vi "GetUnmodifiedSerializableData.vi"(8 "error in (no error)":errorcluster, 11 "BlueSerializable in":refnum<class "BlueSerializable.lvclass">) -> (0 "error out":errorcluster, 2 "SerializableData (parent,child)":variant[](array[variant]), 3 "BlueSerializable out":refnum<class "BlueSerializable.lvclass">)   [LabVIEW 2020, in "BlueSerialization.lvlib" / "BlueSerializer.lvclass"]
uses:
  BlueSerializer.lvclass
  BlueSerializable/BlueSerializable.lvclass
  SerializeOptionsPayload.ctl
  SerializeOptions.ctl
  ClassNameCacheMap.ctl
  ClassNameObj.ctl
  GetSerializableDataAction.ctl
  Support/GetSerializableDataCluster.ctl
  Support/GetSerializableDataClusterClass.ctl
  Support/SerializableDataGetDataAction.ctl
  ClassNameAndVersion.ctl
  <vilib>/Utility/EditLVLibs/LibVersion.ctl
  <vilib>/Utility/EditLVLibs/Edit LVLibs.lvlib
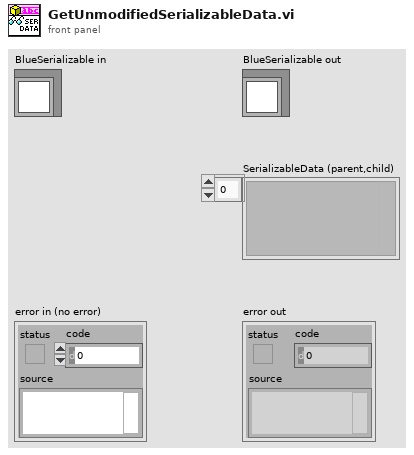
[diagram p1: front panel]
types:
  T1 = typedef "BlueSerialization.lvlib/BlueSerializer.lvclass/SerializeOptionsPayload.ctl" = cluster{"Serialize":T2, "ClassName Cache":refnum<data-value>}
  T2 = typedef "BlueSerialization.lvlib/BlueSerializer.lvclass/SerializeOptions.ctl" = cluster{"serialize non-BlueSerializable objects as hex?":bool, "slice objects per SetSerializeSliceClass.vi?":bool}
  T3 = typedef "BlueSerialization.lvlib/BlueSerializer.lvclass/GetSerializableDataAction.ctl" = enum16{"Ready For Flatten", "Unmodified Data Access"}
  T4 = typedef "BlueSerialization.lvlib/BlueSerializer.lvclass/GetSerializableDataCluster.ctl" = cluster{"Run-Mode":T3, "ClassOps":T5[], "Data":variant[], "PlaceholderData?":bool[]}
  T5 = typedef "BlueSerialization.lvlib/BlueSerializer.lvclass/GetSerializableDataClusterClass.ctl" = cluster{"Action":T6, "Class":T7}
  T6 = typedef "BlueSerialization.lvlib/BlueSerializer.lvclass/SerializableDataGetDataAction.ctl" = enum16{"Add Class", "Drop Class"}
  T7 = typedef "BlueSerialization.lvlib/BlueSerializer.lvclass/ClassNameAndVersion.ctl" = cluster{"class name":string, "Class Version":T8}
  T8 = typedef "Edit LVLibs.lvlib/LibVersion.ctl" = cluster{"Major":u16, "Minor":u16, "Fix":u16, "Build":u16}
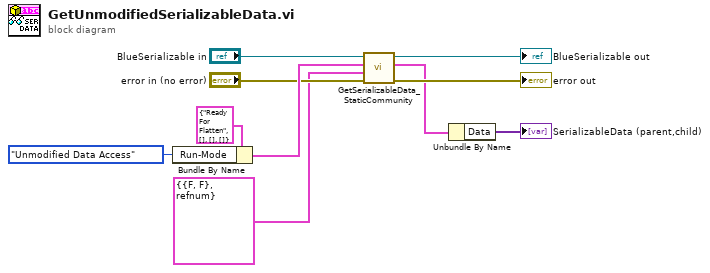
[diagram p0: block diagram]
diagram:
  n1 = Bundle By Name(cluster=T4 {"Run-Mode"=enum."Ready For Flatten", "ClassOps"=[], "Data"=[], "PlaceholderData?"=[]} ("MyData"), "Run-Mode"=GetSerializableDataAction."Unmodified Data Access") -> (w9:T4)
  n2 = call "GetSerializableData_StaticCommunity.vi"("error in (no error)"="error in (no error)", "Options"=T1 {"Serialize"={"serialize non-BlueSerializable objects as hex?"=FALSE, "slice objects per SetSerializeSliceClass.vi?"=FALSE}, "ClassName Cache"=refnum}, "Data in"=w9, "BlueSerializable in"="BlueSerializable in") -> ("error out"=→"error out":errorcluster, "Data out"=w2:T4, "BlueSerializable out"=→"BlueSerializable out":refnum<class "BlueSerializable.lvclass">)  [unwired: 5 in]
  n3 = Unbundle By Name(w2) -> ("Data"=→"SerializableData (parent,child)":variant[])
